vi "Load Becker-Hickl Measurement Descriptions.vi"(6 "Measurement Description Length":i16 format="%.0x", 8 "Error In":errorcluster, 9 "# Measurement Description Blocks":i16 format="%.0x", 10 "Measurement Description Block Offset":i32, 11 "File Path Control":path) -> (0 "Error Out":errorcluster, 2 "Measurement Information":T1 {"Measurement FCS Info"."FCS Type" format="%.0b"; "Measurement FCS Info"."FCS Decay Calc" format="%016b"; "Measurement Stop Info"."Flags" format="%016b"}, 3 "File Path":path)   [LabVIEW 2021, in "Becker-Hickl Files.lvlib"]
uses:
  Becker-Hickl Files.lvlib
  Becker-Hickl Measurement Information.ctl
  Becker-Hickl Measurement Stop Info.ctl
  Becker-Hickl FCS Measurement Info.ctl
  Becker-Hickl Additional Histogram Measurement Info.ctl
  Becker-Hickl Read Single I16.vi
  Becker-Hickl Read Single U16.vi
  Becker-Hickl Read Single U8.vi
  Becker-Hickl Read Single I32.vi
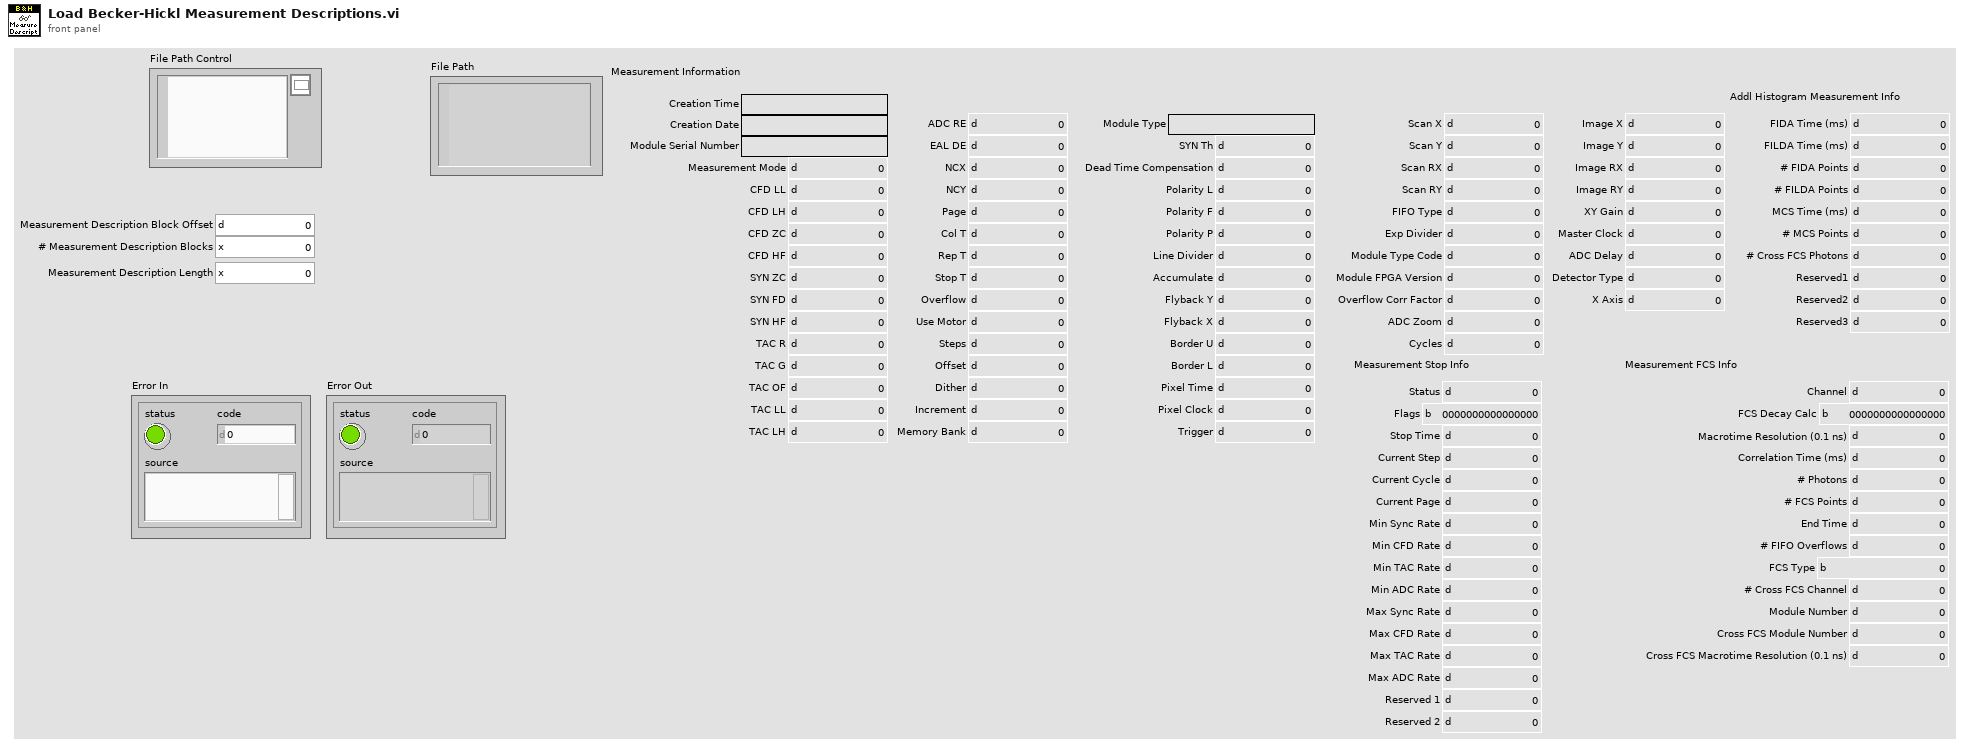
[diagram p1: front panel]
types:
  T1 = typedef "Becker-Hickl Files.lvlib/Becker-Hickl Measurement Information.ctl" = cluster{"Measurement Stop Info":T2, "Measurement FCS Info":T3, "Addl Histogram Measurement Info":T4, "Creation Time":string, "Creation Date":string, "Module Serial Number":string, "Measurement Mode":i16, "CFD LL":sgl, "CFD LH":sgl, "CFD ZC":sgl, "CFD HF":sgl, "SYN ZC":sgl, "SYN FD":i16, "SYN HF":sgl, "TAC R":sgl, "TAC G":i16, "TAC OF":sgl, "TAC LL":sgl, "TAC LH":sgl, "ADC RE":i16, "EAL DE":i16, "NCX":i16, "NCY":i16, "Page":u16, "Col T":sgl, "Rep T":sgl, "Stop T":i16, "Overflow":u8, "Use Motor":i16, "Steps":u16, "Offset":sgl, "Dither":i16, "Increment":i16, "Memory Bank":i16, "Module Type":string, "SYN Th":sgl, "Dead Time Compensation":i16, "Polarity L":i16, "Polarity F":i16, "Polarity P":i16, "Line Divider":i16, "Accumulate":i16, "Flyback Y":i32, "Flyback X":i32, "Border U":i32, "Border L":i32, "Pixel Time":sgl, "Pixel Clock":i16, "Trigger":i16, "Scan X":i32, "Scan Y":i32, "Scan RX":i32, "Scan RY":i32, "FIFO Type":i16, "Exp Divider":i32, "Module Type Code":u16, "Module FPGA Version":u16, "Overflow Corr Factor":sgl, "ADC Zoom":i32, "Cycles":i32, "Image X":i32, "Image Y":i32, "Image RX":i32, "Image RY":i32, "XY Gain":i16, "Master Clock":i16, "ADC Delay":i16, "Detector Type":i16, "X Axis":i16}
  T2 = typedef "Becker-Hickl Files.lvlib/Becker-Hickl Measurement Stop Info.ctl" = cluster{"Status":u16, "Flags":u16, "Stop Time":sgl, "Current Step":i32, "Current Cycle":i32, "Current Page":i32, "Min Sync Rate":sgl, "Min CFD Rate":sgl, "Min TAC Rate":sgl, "Min ADC Rate":sgl, "Max Sync Rate":sgl, "Max CFD Rate":sgl, "Max TAC Rate":sgl, "Max ADC Rate":sgl, "Reserved 1":i32, "Reserved 2":sgl}
  T3 = typedef "Becker-Hickl Files.lvlib/Becker-Hickl FCS Measurement Info.ctl" = cluster{"Channel":u16, "FCS Decay Calc":u16, "Macrotime Resolution (0.1 ns)":u32, "Correlation Time (ms)":sgl, "# Photons":u32, "# FCS Points":i32, "End Time":sgl, "# FIFO Overflows":u16, "FCS Type":u16, "# Cross FCS Channel":u16, "Module Number":u16, "Cross FCS Module Number":u16, "Cross FCS Macrotime Resolution (0.1 ns)":u32}
  T4 = typedef "Becker-Hickl Files.lvlib/Becker-Hickl Additional Histogram Measurement Info.ctl" = cluster{"FIDA Time (ms)":sgl, "FILDA Time (ms)":sgl, "# FIDA Points":i32, "# FILDA Points":i32, "MCS Time (ms)":sgl, "# MCS Points":i32, "# Cross FCS Photons":u32, "Reserved1":i32, "Reserved2":dbl, "Reserved3":dbl}
  T5 = enum16{"time", "date", "mod_ser_no", "meas_mode", "cfd_ll", "cfd_lh", "cfd_zc", "cfd_hf", "syn_zc", "syn_fd", "syn_hf", "tac_r", "tac_g", "tac_of", "tac_ll", "tac_lh", "adc_re", "eal_de", "ncx", "ncy", "page", "col_t", "rep_t", "stopt", "overfl", "use_motor", "steps", "offset", "dither", "incr", "mem_bank", "mod_type", "syn_th", "dead_time_comp", "polarity_l", "polarity_f", "polarity_p", "linediv", "accumulate", "flbck_y", "flbck_x", "bord_u", "bord_l", "pix_time", "pix_clk", "trigger", "scan_x", "scan_y", "scan_rx", "scan_ry", "fifo_typ", "epx_div", "mod_type_code", "mod_fpga_ver", "overflow_corr_factor", "adc_zoom", "cycles", "StopInfo", "FCSInfo", "image_x", "image_y", "image_rx", "image_ry", "xy_gain", "master_clock", "adc_de", "det_type", "x_axis", "HISTInfo"}
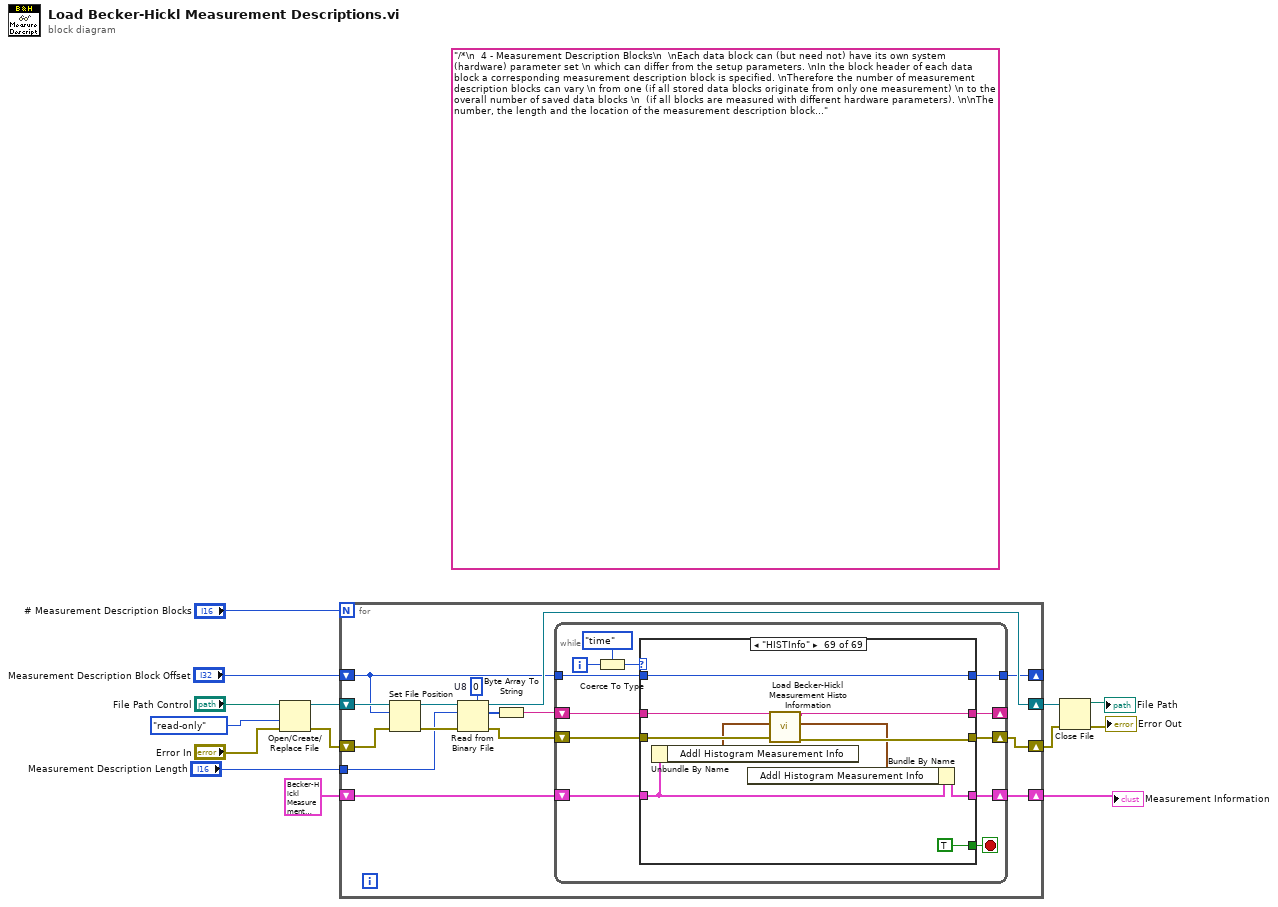
[diagram p0: block diagram]
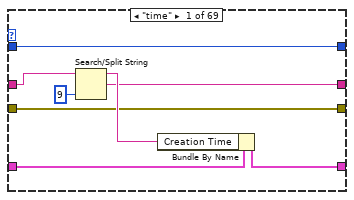
[diagram p2: hidden frame]
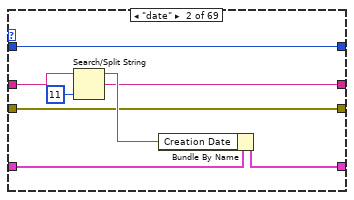
[diagram p3: hidden frame]
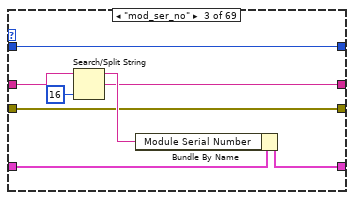
[diagram p4: hidden frame]
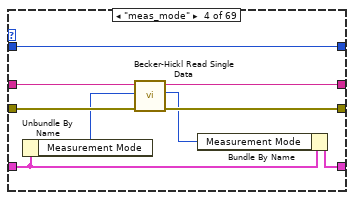
[diagram p5: hidden frame]
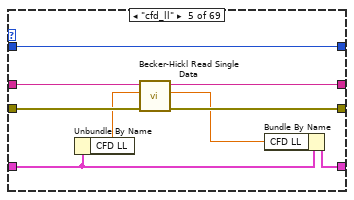
[diagram p6: hidden frame]
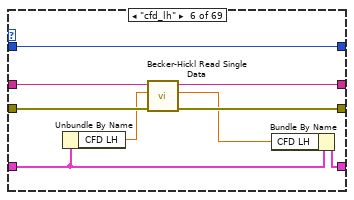
[diagram p7: hidden frame]
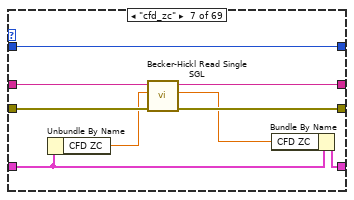
[diagram p8: hidden frame]
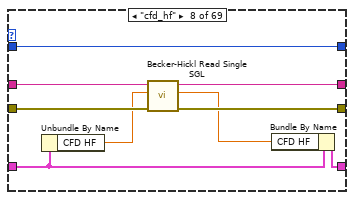
[diagram p9: hidden frame]
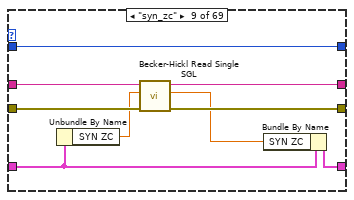
[diagram p10: hidden frame]
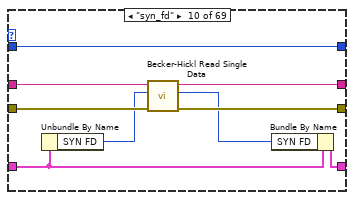
[diagram p11: hidden frame]
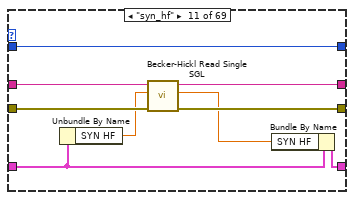
[diagram p12: hidden frame]
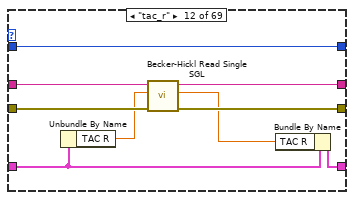
[diagram p13: hidden frame]
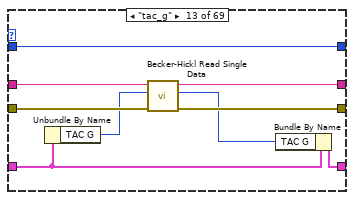
[diagram p14: hidden frame]
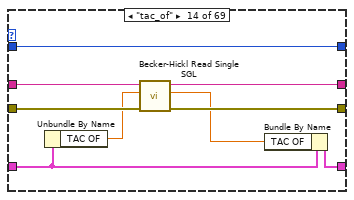
[diagram p15: hidden frame]
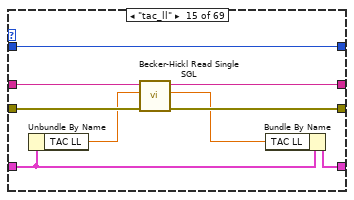
[diagram p16: hidden frame]
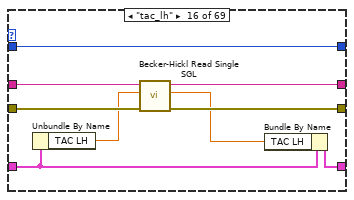
[diagram p17: hidden frame]
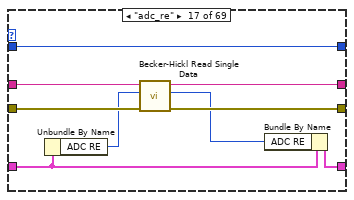
[diagram p18: hidden frame]
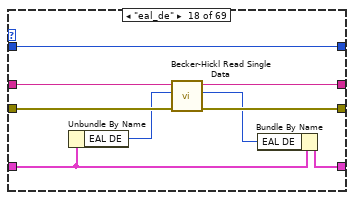
[diagram p19: hidden frame]
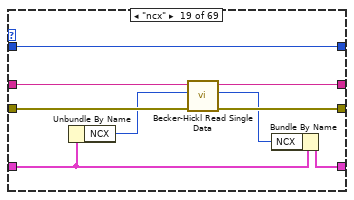
[diagram p20: hidden frame]
diagram:
  (unwired) "/*\n  4 - Measurement Description Blocks\n  \nEach data block can (but need not) have its own system (hardware) parameter set \n which can differ from the setup parameters. \nIn the block header of each data block a corresponding measurement description block is specified. \nTherefore the number of measurement description blocks can vary \n from one (if all stored data blocks originate from only one measurement) \n to the overall number of saved data blocks \n  (if all blocks are measured with different hardware parameters). \n\nThe number, the length and the location of the measurement description blocks is stored \n  in the file header at the beginning of the file.\nThe information in the measurement description blocks is used for \n the 'Block Info' or 'Set Info' function in the Load, Save and Trace Parameters menus. \nIf the button 'Use System Parameters from the Selected Block' is pressed, \n the system parameters are replaced by the data in the measurement description block.\nThe measurement description blocks are stored in a binary format. \n\nFrom the software version 7.9  measurement description block contains also additional \n information (in the structure MeasStopInfo ) collected at the end of the measurement. \n This information can be useful when analyzing system's wrong setup or malfunction.\n\nFrom the software version 8.1  measurement description block contains also additional \n information (in the structure MeasFCSInfo ) collected at the end of the FIFO measurement\n when FCS curve were created.\n The information is valid only for data blocks of type FIFO_DATA or FIFO_DATA_FROM_FILE\n\nFrom the software version 8.3  measurement description block contains also additional \n information (in the structure MeasFIDAInfo ) collected at the end of the FIFO measurement\n when FIDA or FILDA curves were created.\n The information is valid only for data blocks of type FIFO_DATA or FIFO_DATA_FROM_FILE\n\nFrom the software version 8.4  measurement description block contains instead of MeasFIDAInfo\n the structure MeasHISTInfo  collected at the end of the FIFO measurement\n when FIDA , FILDA or MCS curves were created. \n It contains additionally information for MCS curve.\n The information is valid only for data blocks of type FIFO_DATA or FIFO_DATA_FROM_FILE\n\nThe structures are shown below.\n\n*/\n\n\ntypedef struct {\n  unsigned short  status;  // last SPC_test_state return value ( status )\n  unsigned short  flags;   // scan clocks bits 2-0( frame, line, pixel), \n                           //  rates_read - bit 15\n  float  stop_time;        // time from start to  - disarm ( simple measurement )\n                           //    - or to the end of the cycle (for complex measurement )\n  int    cur_step;         // current step  ( if multi-step measurement )\n  int    cur_cycle;        // current cycle (accumulation cycle in FLOW mode ) -\n                           //  ( if multi-cycle measurement ) \n  int    cur_page;         // current measured page\n  float  min_sync_rate;    // minimum rates during the measurement\n  float  min_cfd_rate;     //   ( -1.0 - not set )\n  float  min_tac_rate;\n  float  min_adc_rate;\n  float  max_sync_rate;    // maximum rates during the measurement\n  float  max_cfd_rate;     //   ( -1.0 - not set )\n  float  max_tac_rate;\n  float  max_adc_rate;\n  int    reserved1;\n  float  reserved2;\n  }MeasStopInfo;           // information collected when measurement is finished\n  \n\n\ntypedef struct {\n  unsigned short  chan;               // routing channel number\n  unsigned short  fcs_decay_calc;     // bit 0 = 1 - decay curve calculated\n                                      // bit 1 = 1 - fcs   curve calculated\n                                      // bit 2 = 1 - FIDA  curve calculated\n                                      // bit 3 = 1 - FILDA curve calculated\n                                      // bit 4 = 1 - MCS curve calculated\n                                      // bit 5 = 1 - 3D Image calculated\n  unsigned int    mt_resol;           // macro time clock in 0.1 ns units\n  float           cortime;            // correlation time [ms] \n  unsigned int    calc_photons;       //  no of photons  \n  int             fcs_points;         // no of FCS values\n  float           end_time;           // macro time of the last photon \n  unsigned short  overruns;           // no of Fifo overruns \n                              //   when > 0  fcs curve & end_time are not valid\n  unsigned short  fcs_type;   // 0 - linear FCS with log binning ( 100 bins/log )\n                              // when bit 15 = 1 ( 0x8000 ) - Multi-Tau FCS \n                              //           where bits 14-0 = ktau parameter\n  unsigned short  cross_chan;         // cross FCS routing channel number\n                   //   when chan = cross_chan and mod == cross_mod - Auto FCS\n                   //        otherwise - Cross FCS\n  unsigned short  mod;                // module number\n  unsigned short  cross_mod;          // cross FCS module number\n  unsigned int    cross_mt_resol;     // macro time clock of cross FCS module in 0.1 ns units\n  }MeasFCSInfo;   // information collected when FIFO measurement is finished\n\n\n  \ntypedef struct {\n  float           fida_time;          // interval time [ms] for FIDA histogram\n  float           filda_time;         // interval time [ms] for FILDA histogram\n  int             fida_points;        // no of FIDA values\n                                      //    or current frame number ( fifo_image)\n  int             filda_points;       // no of FILDA values\n                                      //    or current line  number ( fifo_image)\n  float           mcs_time;            // interval time [ms] for MCS histogram\n  int             mcs_points;          // no of MCS values\n                                      //    or current pixel number ( fifo_image)\n  unsigned int    cross_calc_phot;    //  no of calculated photons from cross_channel \n                                      //    for Cross FCS histogram\n  int             reserved1;\n  double          reserved2;\n  double          reserved3;\n  }MeasHISTInfo;     // extension of MeasFCSInfo for other histograms ( FIDA, FILDA, MCS ) \n  \n\ntypedef struct _MeasureInfo {\n  char     time[9];        /* time of creation */\n  char     date[11];       /* date of creation */\n  char     mod_ser_no[16]; /* serial number of the module */\n  short    meas_mode;\n  float    cfd_ll;\n  float    cfd_lh;\n  float    cfd_zc;\n  float    cfd_hf;\n  float    syn_zc;\n  short    syn_fd;\n  float    syn_hf;\n  float    tac_r;\n  short    tac_g;\n  float    tac_of;\n  float    tac_ll;\n  float    tac_lh;\n  short    adc_re;\n  short    eal_de;\n  short    ncx;\n  short    ncy;\n  unsigned short  page;\n  float    col_t;\n  float    rep_t;\n  short    stopt;\n  char     overfl;\n  short    use_motor;\n  unsigned short    steps;\n  float    offset;\n  short    dither;\n  short    incr;\n  short    mem_bank;\n  char     mod_type[16];   /* module type */\n  float    syn_th;\n  short    dead_time_comp;\n  short    polarity_l;   //  2 = disabled line markers\n  short    polarity_f;\n  short    polarity_p;\n  short    linediv;      // line predivider = 2 ** ( linediv)\n  short    accumulate;\n  int      flbck_y; \n  int      flbck_x; \n  int      bord_u; \n  int      bord_l; \n  float    pix_time;\n  short    pix_clk; \n  short    trigger; \n  int      scan_x; \n  int      scan_y; \n  int      scan_rx; \n  int      scan_ry; \n  short    fifo_typ;\n  int      epx_div; \n  unsigned short  mod_type_code; \n  unsigned short  mod_fpga_ver;    // new in v.8.4\n  float    overflow_corr_factor;\n  int      adc_zoom; \n  int      cycles;        //  cycles ( accumulation cycles in FLOW mode ) \n  MeasStopInfo StopInfo;\n  MeasFCSInfo  FCSInfo;   // valid only for FIFO meas\n  int      image_x;       // 4 subsequent fields valid only for Camera mode\n  int      image_y;       //     or FIFO_IMAGE mode\n  int      image_rx; \n  int      image_ry; \n  short    xy_gain;       // gain for XY ADCs ( SPC930 )\n  short    master_clock;  // use or not  Master Clock (SPC140 multi-module )\n  short    adc_de;        // ADC sample delay ( SPC-930 )\n  short    det_type;      // detector type ( SPC-930 in camera mode ) \n  short    x_axis;        // X axis representation ( SPC-930 ) \n  MeasHISTInfo  HISTInfo; // extension of FCSInfo, valid only for FIFO meas\n  }MeasureInfo;\n\n"
  n1 = Open/Create/Replace File(file path (use dialog)="File Path Control", error in="Error In", access (0:read/write)=enum16{"read/write", "read-only", "write-only"}."read-only") -> (refnum out=w11:refnum<file>, error out=w10:errorcluster)  [unwired: 3 in, 1 out]
  n2 = for {
    N: "# Measurement Description Blocks" -> [_]
    shift-right: [w23] -> w7
    shift-left: w10 -> [w26]
    shift-right: [w21] -> w8
    shift-left: w11 -> [w27]
    shift-right: [w20] -> _
    shift-left: "Measurement Description Block Offset" -> [w19]
    tunnel: "Measurement Description Length" -> [w18]
    shift-right: [w16] -> w1
    shift-left: T1 {"Measurement Stop Info"={"Status"=0, "Flags"=0, "Stop Time"=0.0, "Current Step"=0, "Current Cycle"=0, "Current Page"=0, "Min Sync Rate"=0.0, "Min CFD Rate"=0.0, "Min TAC Rate"=0.0, "Min ADC Rate"=0.0, "Max Sync Rate"=0.0, "Max CFD Rate"=0.0, "Max TAC Rate"=0.0, "Max ADC Rate"=0.0, "Reserved 1"=0, "Reserved 2"=0.0}, "Measurement FCS Info"={"Channel"=0, "FCS Decay Calc"=0, "Macrotime Resolution (0.1 ns)"=0, "Correlation Time (ms)"=0.0, "# Photons"=0, "# FCS Points"=0, "End Time"=0.0, "# FIFO Overflows"=0, "FCS Type"=0, "# Cross FCS Channel"=0, "Module Number"=0, "Cross FCS Module Number"=0, "Cross FCS Macrotime Resolution (0.1 ns)"=0}, "Addl Histogram Measurement Info"={"FIDA Time (ms)"=0.0, "FILDA Time (ms)"=0.0, "# FIDA Points"=0, "# FILDA Points"=0, "MCS Time (ms)"=0.0, "# MCS Points"=0, "# Cross FCS Photons"=0, "Reserved1"=0, "Reserved2"=0.0, "Reserved3"=0.0}, "Creation Time"="", "Creation Date"="", "Module Serial Number"="", "Measurement Mode"=0, "CFD LL"=0.0, "CFD LH"=0.0, "CFD ZC"=0.0, "CFD HF"=0.0, "SYN ZC"=0.0, "SYN FD"=0, "SYN HF"=0.0, "TAC R"=0.0, "TAC G"=0, "TAC OF"=0.0, "TAC LL"=0.0, "TAC LH"=0.0, "ADC RE"=0, "EAL DE"=0, "NCX"=0, "NCY"=0, "Page"=0, "Col T"=0.0, "Rep T"=0.0, "Stop T"=0, "Overflow"=0, "Use Motor"=0, "Steps"=0, "Offset"=0.0, "Dither"=0, "Increment"=0, "Memory Bank"=0, "Module Type"="", "SYN Th"=0.0, "Dead Time Compensation"=0, "Polarity L"=0, "Polarity F"=0, "Polarity P"=0, "Line Divider"=0, "Accumulate"=0, "Flyback Y"=0, "Flyback X"=0, "Border U"=0, "Border L"=0, "Pixel Time"=0.0, "Pixel Clock"=0, "Trigger"=0, "Scan X"=0, "Scan Y"=0, "Scan RX"=0, "Scan RY"=0, "FIFO Type"=0, "Exp Divider"=0, "Module Type Code"=0, "Module FPGA Version"=0, "Overflow Corr Factor"=0.0, "ADC Zoom"=0, "Cycles"=0, "Image X"=0, "Image Y"=0, "Image RX"=0, "Image RY"=0, "XY Gain"=0, "Master Clock"=0, "ADC Delay"=0, "Detector Type"=0, "X Axis"=0} ("Measurement Information") -> [w17]
    w29 = u8 0  # U8
    n3 = Set File Position(offset (in bytes) (0)=w19, refnum=w27, error in=w26) -> (refnum out=w25:refnum<file>, error out=w24:errorcluster)  [unwired: 1 in]
    n4 = Read from Binary File(5:w29, 8:w24, 10:w18, 11:w25) -> (0:w22:errorcluster, 2:w28:u8[], 3:w21:refnum<file>)  [unwired: 2 in, 1 out]
    n5 = Byte Array To String(unsigned byte array=w28) -> (string=w15:string)
    n6 = while {
      shift-right: [w36] -> w23
      shift-left: w22 -> [w40]
      shift-right: [w35] -> _
      shift-left: w15 -> [w39]
      shift-right: [w37] -> w16
      shift-left: w17 -> [w38]
      tunnel: [w34] -> w20
      tunnel: w19 -> [w33]
      i -> [w41]
      stop <- w30 stop-if-true
      n7 = Coerce To Type(0:w41, 1:T5."time") -> (2:w32:T5)
      n8 = case shown="\"HISTInfo\"" w32 {
        tunnel: w40 -> [w42 w50 w58 w71 w80 w89 w98 w107 w116 w125 w134 w143 w152 w161 w170 w179 w188 w197 w206 w215 w224 w233 w242 w251 w260 w269 w278 w287 w296 w305 w314 w321 w331 w340 w349 w358 w367 w376 w385 w394 w403 w412 w421 w430 w439 w448 w457 w466 w475 w484 w493 w502 w511 w520 w529 w538 w547 w554 w563 w574 w583 w592 w601 w610 w619 w628 w637 w646 w654]
        tunnel: w39 -> [w46 w54 w62 w72 w81 w90 w99 w108 w117 w126 w135 w144 w153 w162 w171 w180 w189 w198 w207 w216 w225 w234 w243 w252 w261 w270 w279 w288 w297 w306 w315 w322 w332 w341 w350 w359 w368 w377 w386 w395 w404 w413 w422 w431 w440 w449 w458 w467 w476 w485 w494 w503 w512 w521 w530 w539 w548 w556 w565 w575 w584 w593 w602 w611 w620 w629 w638 w647 w655]
        tunnel: w38 -> [w48 w56 w64 w67 w76 w85 w94 w103 w112 w121 w130 w139 w148 w157 w166 w175 w184 w193 w202 w211 w220 w229 w238 w247 w256 w265 w274 w283 w292 w301 w310 w323 w327 w336 w345 w354 w363 w372 w381 w390 w399 w408 w417 w426 w435 w444 w453 w462 w471 w480 w489 w498 w507 w516 w525 w534 w543 w557 w566 w570 w579 w588 w597 w606 w615 w624 w633 w642 w657]
        tunnel: [w47 w55 w63 w73 w82 w91 w100 w109 w118 w127 w136 w145 w154 w163 w172 w181 w190 w199 w208 w217 w226 w235 w244 w253 w262 w271 w280 w289 w298 w307 w316 w324 w333 w342 w351 w360 w369 w378 w387 w396 w405 w414 w423 w432 w441 w450 w459 w468 w477 w486 w495 w504 w513 w522 w531 w540 w549 w558 w567 w576 w585 w594 w603 w612 w621 w630 w639 w648 w658] -> w37
        tunnel: [w42 w50 w58 w70 w79 w88 w97 w106 w115 w124 w133 w142 w151 w160 w169 w178 w187 w196 w205 w214 w223 w232 w241 w250 w259 w268 w277 w286 w295 w304 w313 w321 w330 w339 w348 w357 w366 w375 w384 w393 w402 w411 w420 w429 w438 w447 w456 w465 w474 w483 w492 w501 w510 w519 w528 w537 w546 w553 w562 w573 w582 w591 w600 w609 w618 w627 w636 w645 w652] -> w36
        tunnel: [w43 w51 w59 w69 w78 w87 w96 w105 w114 w123 w132 w141 w150 w159 w168 w177 w186 w195 w204 w213 w222 w231 w240 w249 w258 w267 w276 w285 w294 w303 w312 w319 w329 w338 w347 w356 w365 w374 w383 w392 w401 w410 w419 w428 w437 w446 w455 w464 w473 w482 w491 w500 w509 w518 w527 w536 w545 w555 w564 w572 w581 w590 w599 w608 w617 w626 w635 w644 w653] -> w35
        tunnel: [w49 w57 w65 w74 w83 w92 w101 w110 w119 w128 w137 w146 w155 w164 w173 w182 w191 w200 w209 w218 w227 w236 w245 w254 w263 w272 w281 w290 w299 w308 w317 w325 w334 w343 w352 w361 w370 w379 w388 w397 w406 w415 w424 w433 w442 w451 w460 w469 w478 w487 w496 w505 w514 w523 w532 w541 w550 w559 w568 w577 w586 w595 w604 w613 w622 w631 w640 w649 w659] -> w34
        tunnel: w33 -> [w49 w57 w65 w74 w83 w92 w101 w110 w119 w128 w137 w146 w155 w164 w173 w182 w191 w200 w209 w218 w227 w236 w245 w254 w263 w272 w281 w290 w299 w308 w317 w325 w334 w343 w352 w361 w370 w379 w388 w397 w406 w415 w424 w433 w442 w451 w460 w469 w478 w487 w496 w505 w514 w523 w532 w541 w550 w559 w568 w577 w586 w595 w604 w613 w622 w631 w640 w649 w659]
        tunnel: [_ _ _ _ _ _ _ _ _ _ _ _ _ _ _ _ _ _ _ _ _ _ _ _ _ _ _ _ _ _ _ _ _ _ _ _ _ _ _ _ _ _ _ _ _ _ _ _ _ _ _ _ _ _ _ _ _ _ _ _ _ _ _ _ _ _ _ _ TRUE] -> w30
        frame "time" {
          n9 = Search/Split String(string=w46, offset (0)=9) -> (substring before match=w44:string, match + rest of string=w43:string)  [unwired: 1 in, 1 out]
          n10 = Bundle By Name(cluster=w48, "Creation Time"=w44) -> (w47:T1)
        }
        frame "date" {
          n11 = Search/Split String(string=w54, offset (0)=11) -> (substring before match=w52:string, match + rest of string=w51:string)  [unwired: 1 in, 1 out]
          n12 = Bundle By Name(cluster=w56, "Creation Date"=w52) -> (w55:T1)
        }
        frame "mod_ser_no" {
          n13 = Search/Split String(string=w62, offset (0)=16) -> (substring before match=w60:string, match + rest of string=w59:string)  [unwired: 1 in, 1 out]
          n14 = Bundle By Name(cluster=w64, "Module Serial Number"=w60) -> (w63:T1)
        }
        frame "meas_mode" {
          n15 = Unbundle By Name(w67) -> ("Measurement Mode"=w66:i16)
          n16 = call-poly "Becker-Hickl Read Single Data.vi"("Error In"=w71, "Default"=w66, "Bytes in"=w72) -> ("Error Out"=w70:errorcluster, "I16"=w68:i16, "Bytes out"=w69:string)  [unwired: 6 in]
          n17 = Bundle By Name(cluster=w67, "Measurement Mode"=w68) -> (w73:T1)
        }
        frame "cfd_ll" {
          n18 = Unbundle By Name(w76) -> ("CFD LL"=w75:sgl)
          n19 = call-poly "Becker-Hickl Read Single Data.vi"("Error In"=w80, "Default"=w75, "Bytes in"=w81) -> ("Error Out"=w79:errorcluster, "SGL"=w77:sgl, "Bytes out"=w78:string)  [unwired: 6 in]
          n20 = Bundle By Name(cluster=w76, "CFD LL"=w77) -> (w82:T1)
        }
        frame "cfd_lh" {
          n21 = Unbundle By Name(w85) -> ("CFD LH"=w84:sgl)
          n22 = call-poly "Becker-Hickl Read Single Data.vi"("Error In"=w89, "Default"=w84, "Bytes in"=w90) -> ("Error Out"=w88:errorcluster, "SGL"=w86:sgl, "Bytes out"=w87:string)  [unwired: 6 in]
          n23 = Bundle By Name(cluster=w85, "CFD LH"=w86) -> (w91:T1)
        }
        frame "cfd_zc" {
          n24 = Unbundle By Name(w94) -> ("CFD ZC"=w93:sgl)
          n25 = call "Becker-Hickl Read Single SGL.vi"("Error In"=w98, "Default"=w93, "Bytes in"=w99) -> ("Error Out"=w97:errorcluster, "SGL"=w95:sgl, "Bytes out"=w96:string)  [unwired: 6 in]
          n26 = Bundle By Name(cluster=w94, "CFD ZC"=w95) -> (w100:T1)
        }
        frame "cfd_hf" {
          n27 = Unbundle By Name(w103) -> ("CFD HF"=w102:sgl)
          n28 = call "Becker-Hickl Read Single SGL.vi"("Error In"=w107, "Default"=w102, "Bytes in"=w108) -> ("Error Out"=w106:errorcluster, "SGL"=w104:sgl, "Bytes out"=w105:string)  [unwired: 6 in]
          n29 = Bundle By Name(cluster=w103, "CFD HF"=w104) -> (w109:T1)
        }
        frame "syn_zc" {
          n30 = Unbundle By Name(w112) -> ("SYN ZC"=w111:sgl)
          n31 = call "Becker-Hickl Read Single SGL.vi"("Error In"=w116, "Default"=w111, "Bytes in"=w117) -> ("Error Out"=w115:errorcluster, "SGL"=w113:sgl, "Bytes out"=w114:string)  [unwired: 6 in]
          n32 = Bundle By Name(cluster=w112, "SYN ZC"=w113) -> (w118:T1)
        }
        frame "syn_fd" {
          n33 = Unbundle By Name(w121) -> ("SYN FD"=w120:i16)
          n34 = call-poly "Becker-Hickl Read Single Data.vi"("Error In"=w125, "Default"=w120, "Bytes in"=w126) -> ("Error Out"=w124:errorcluster, "I16"=w122:i16, "Bytes out"=w123:string)  [unwired: 6 in]
          n35 = Bundle By Name(cluster=w121, "SYN FD"=w122) -> (w127:T1)
        }
        frame "syn_hf" {
          n36 = Unbundle By Name(w130) -> ("SYN HF"=w129:sgl)
          n37 = call "Becker-Hickl Read Single SGL.vi"("Error In"=w134, "Default"=w129, "Bytes in"=w135) -> ("Error Out"=w133:errorcluster, "SGL"=w131:sgl, "Bytes out"=w132:string)  [unwired: 6 in]
          n38 = Bundle By Name(cluster=w130, "SYN HF"=w131) -> (w136:T1)
        }
        frame "tac_r" {
          n39 = Unbundle By Name(w139) -> ("TAC R"=w138:sgl)
          n40 = call "Becker-Hickl Read Single SGL.vi"("Error In"=w143, "Default"=w138, "Bytes in"=w144) -> ("Error Out"=w142:errorcluster, "SGL"=w140:sgl, "Bytes out"=w141:string)  [unwired: 6 in]
          n41 = Bundle By Name(cluster=w139, "TAC R"=w140) -> (w145:T1)
        }
        frame "tac_g" {
          n42 = Unbundle By Name(w148) -> ("TAC G"=w147:i16)
          n43 = call-poly "Becker-Hickl Read Single Data.vi"("Error In"=w152, "Default"=w147, "Bytes in"=w153) -> ("Error Out"=w151:errorcluster, "I16"=w149:i16, "Bytes out"=w150:string)  [unwired: 6 in]
          n44 = Bundle By Name(cluster=w148, "TAC G"=w149) -> (w154:T1)
        }
        frame "tac_of" {
          n45 = Unbundle By Name(w157) -> ("TAC OF"=w156:sgl)
          n46 = call "Becker-Hickl Read Single SGL.vi"("Error In"=w161, "Default"=w156, "Bytes in"=w162) -> ("Error Out"=w160:errorcluster, "SGL"=w158:sgl, "Bytes out"=w159:string)  [unwired: 6 in]
          n47 = Bundle By Name(cluster=w157, "TAC OF"=w158) -> (w163:T1)
        }
        frame "tac_ll" {
          n48 = Unbundle By Name(w166) -> ("TAC LL"=w165:sgl)
          n49 = call "Becker-Hickl Read Single SGL.vi"("Error In"=w170, "Default"=w165, "Bytes in"=w171) -> ("Error Out"=w169:errorcluster, "SGL"=w167:sgl, "Bytes out"=w168:string)  [unwired: 6 in]
          n50 = Bundle By Name(cluster=w166, "TAC LL"=w167) -> (w172:T1)
        }
        frame "tac_lh" {
          n51 = Unbundle By Name(w175) -> ("TAC LH"=w174:sgl)
          n52 = call "Becker-Hickl Read Single SGL.vi"("Error In"=w179, "Default"=w174, "Bytes in"=w180) -> ("Error Out"=w178:errorcluster, "SGL"=w176:sgl, "Bytes out"=w177:string)  [unwired: 6 in]
          n53 = Bundle By Name(cluster=w175, "TAC LH"=w176) -> (w181:T1)
        }
        frame "adc_re" {
          n54 = Unbundle By Name(w184) -> ("ADC RE"=w183:i16)
          n55 = call-poly "Becker-Hickl Read Single Data.vi"("Error In"=w188, "Default"=w183, "Bytes in"=w189) -> ("Error Out"=w187:errorcluster, "I16"=w185:i16, "Bytes out"=w186:string)  [unwired: 6 in]
          n56 = Bundle By Name(cluster=w184, "ADC RE"=w185) -> (w190:T1)
        }
        frame "eal_de" {
          n57 = Unbundle By Name(w193) -> ("EAL DE"=w192:i16)
          n58 = call-poly "Becker-Hickl Read Single Data.vi"("Error In"=w197, "Default"=w192, "Bytes in"=w198) -> ("Error Out"=w196:errorcluster, "I16"=w194:i16, "Bytes out"=w195:string)  [unwired: 6 in]
          n59 = Bundle By Name(cluster=w193, "EAL DE"=w194) -> (w199:T1)
        }
        frame "ncx" {
          n60 = Unbundle By Name(w202) -> ("NCX"=w201:i16)
          n61 = call-poly "Becker-Hickl Read Single Data.vi"("Error In"=w206, "Default"=w201, "Bytes in"=w207) -> ("Error Out"=w205:errorcluster, "I16"=w203:i16, "Bytes out"=w204:string)  [unwired: 6 in]
          n62 = Bundle By Name(cluster=w202, "NCX"=w203) -> (w208:T1)
        }
        frame "ncy" {
          n63 = Unbundle By Name(w211) -> ("NCY"=w210:i16)
          n64 = call-poly "Becker-Hickl Read Single Data.vi"("Error In"=w215, "Default"=w210, "Bytes in"=w216) -> ("Error Out"=w214:errorcluster, "I16"=w212:i16, "Bytes out"=w213:string)  [unwired: 6 in]
          n65 = Bundle By Name(cluster=w211, "NCY"=w212) -> (w217:T1)
        }
        frame "page" {
          n66 = Unbundle By Name(w220) -> ("Page"=w219:u16)
          n67 = call-poly "Becker-Hickl Read Single Data.vi"("Error In"=w224, "Default"=w219, "Bytes in"=w225) -> ("Error Out"=w223:errorcluster, "U16"=w221:u16, "Bytes out"=w222:string)  [unwired: 6 in]
          n68 = Bundle By Name(cluster=w220, "Page"=w221) -> (w226:T1)
        }
        frame "col_t" {
          n69 = Unbundle By Name(w229) -> ("Col T"=w228:sgl)
          n70 = call "Becker-Hickl Read Single SGL.vi"("Error In"=w233, "Default"=w228, "Bytes in"=w234) -> ("Error Out"=w232:errorcluster, "SGL"=w230:sgl, "Bytes out"=w231:string)  [unwired: 6 in]
          n71 = Bundle By Name(cluster=w229, "Col T"=w230) -> (w235:T1)
        }
        frame "rep_t" {
          n72 = Unbundle By Name(w238) -> ("Rep T"=w237:sgl)
          n73 = call "Becker-Hickl Read Single SGL.vi"("Error In"=w242, "Default"=w237, "Bytes in"=w243) -> ("Error Out"=w241:errorcluster, "SGL"=w239:sgl, "Bytes out"=w240:string)  [unwired: 6 in]
          n74 = Bundle By Name(cluster=w238, "Rep T"=w239) -> (w244:T1)
        }
        frame "stopt" {
          n75 = Unbundle By Name(w247) -> ("Stop T"=w246:i16)
          n76 = call-poly "Becker-Hickl Read Single Data.vi"("Error In"=w251, "Default"=w246, "Bytes in"=w252) -> ("Error Out"=w250:errorcluster, "I16"=w248:i16, "Bytes out"=w249:string)  [unwired: 6 in]
          n77 = Bundle By Name(cluster=w247, "Stop T"=w248) -> (w253:T1)
        }
        frame "overfl" {
          n78 = Unbundle By Name(w256) -> ("Overflow"=w255:u8)
          n79 = call-poly "Becker-Hickl Read Single Data.vi"("Error In"=w260, "Default"=w255, "Bytes in"=w261) -> ("Error Out"=w259:errorcluster, "U8"=w257:u8, "Bytes out"=w258:string)  [unwired: 6 in]
          n80 = Bundle By Name(cluster=w256, "Overflow"=w257) -> (w262:T1)
        }
        frame "use_motor" {
          n81 = Unbundle By Name(w265) -> ("Use Motor"=w264:i16)
          n82 = call-poly "Becker-Hickl Read Single Data.vi"("Error In"=w269, "Default"=w264, "Bytes in"=w270) -> ("Error Out"=w268:errorcluster, "I16"=w266:i16, "Bytes out"=w267:string)  [unwired: 6 in]
          n83 = Bundle By Name(cluster=w265, "Use Motor"=w266) -> (w271:T1)
        }
        frame "steps" {
          n84 = Unbundle By Name(w274) -> ("Steps"=w273:u16)
          n85 = call-poly "Becker-Hickl Read Single Data.vi"("Error In"=w278, "Default"=w273, "Bytes in"=w279) -> ("Error Out"=w277:errorcluster, "U16"=w275:u16, "Bytes out"=w276:string)  [unwired: 6 in]
          n86 = Bundle By Name(cluster=w274, "Steps"=w275) -> (w280:T1)
        }
        frame "offset" {
          n87 = Unbundle By Name(w283) -> ("Offset"=w282:sgl)
          n88 = call-poly "Becker-Hickl Read Single Data.vi"("Error In"=w287, "Default"=w282, "Bytes in"=w288) -> ("Error Out"=w286:errorcluster, "SGL"=w284:sgl, "Bytes out"=w285:string)  [unwired: 6 in]
          n89 = Bundle By Name(cluster=w283, "Offset"=w284) -> (w289:T1)
        }
        frame "dither" {
          n90 = Unbundle By Name(w292) -> ("Dither"=w291:i16)
          n91 = call-poly "Becker-Hickl Read Single Data.vi"("Error In"=w296, "Default"=w291, "Bytes in"=w297) -> ("Error Out"=w295:errorcluster, "I16"=w293:i16, "Bytes out"=w294:string)  [unwired: 6 in]
          n92 = Bundle By Name(cluster=w292, "Dither"=w293) -> (w298:T1)
        }
        frame "incr" {
          n93 = Unbundle By Name(w301) -> ("Increment"=w300:i16)
          n94 = call-poly "Becker-Hickl Read Single Data.vi"("Error In"=w305, "Default"=w300, "Bytes in"=w306) -> ("Error Out"=w304:errorcluster, "I16"=w302:i16, "Bytes out"=w303:string)  [unwired: 6 in]
          n95 = Bundle By Name(cluster=w301, "Increment"=w302) -> (w307:T1)
        }
        frame "mem_bank" {
          n96 = Unbundle By Name(w310) -> ("Memory Bank"=w309:i16)
          n97 = call-poly "Becker-Hickl Read Single Data.vi"("Error In"=w314, "Default"=w309, "Bytes in"=w315) -> ("Error Out"=w313:errorcluster, "I16"=w311:i16, "Bytes out"=w312:string)  [unwired: 6 in]
          n98 = Bundle By Name(cluster=w310, "Memory Bank"=w311) -> (w316:T1)
        }
        frame "mod_type" {
          n99 = Search/Split String(string=w322, offset (0)=16) -> (substring before match=w320:string, match + rest of string=w319:string)  [unwired: 1 in, 1 out]
          n100 = Bundle By Name(cluster=w323, "Module Type"=w320) -> (w324:T1)
        }
        frame "syn_th" {
          n101 = Unbundle By Name(w327) -> ("SYN Th"=w326:sgl)
          n102 = call-poly "Becker-Hickl Read Single Data.vi"("Error In"=w331, "Default"=w326, "Bytes in"=w332) -> ("Error Out"=w330:errorcluster, "SGL"=w328:sgl, "Bytes out"=w329:string)  [unwired: 6 in]
          n103 = Bundle By Name(cluster=w327, "SYN Th"=w328) -> (w333:T1)
        }
        frame "dead_time_comp" {
          n104 = Unbundle By Name(w336) -> ("Dead Time Compensation"=w335:i16)
          n105 = call-poly "Becker-Hickl Read Single Data.vi"("Error In"=w340, "Default"=w335, "Bytes in"=w341) -> ("Error Out"=w339:errorcluster, "I16"=w337:i16, "Bytes out"=w338:string)  [unwired: 6 in]
          n106 = Bundle By Name(cluster=w336, "Dead Time Compensation"=w337) -> (w342:T1)
        }
        frame "polarity_l" {
          n107 = Unbundle By Name(w345) -> ("Polarity L"=w344:i16)
          n108 = call-poly "Becker-Hickl Read Single Data.vi"("Error In"=w349, "Default"=w344, "Bytes in"=w350) -> ("Error Out"=w348:errorcluster, "I16"=w346:i16, "Bytes out"=w347:string)  [unwired: 6 in]
          n109 = Bundle By Name(cluster=w345, "Polarity L"=w346) -> (w351:T1)
        }
        frame "polarity_f" {
          n110 = Unbundle By Name(w354) -> ("Polarity F"=w353:i16)
          n111 = call-poly "Becker-Hickl Read Single Data.vi"("Error In"=w358, "Default"=w353, "Bytes in"=w359) -> ("Error Out"=w357:errorcluster, "I16"=w355:i16, "Bytes out"=w356:string)  [unwired: 6 in]
          n112 = Bundle By Name(cluster=w354, "Polarity F"=w355) -> (w360:T1)
        }
        frame "polarity_p" {
          n113 = Unbundle By Name(w363) -> ("Polarity P"=w362:i16)
          n114 = call-poly "Becker-Hickl Read Single Data.vi"("Error In"=w367, "Default"=w362, "Bytes in"=w368) -> ("Error Out"=w366:errorcluster, "I16"=w364:i16, "Bytes out"=w365:string)  [unwired: 6 in]
          n115 = Bundle By Name(cluster=w363, "Polarity P"=w364) -> (w369:T1)
        }
        frame "linediv" {
          n116 = Unbundle By Name(w372) -> ("Line Divider"=w371:i16)
          n117 = call-poly "Becker-Hickl Read Single Data.vi"("Error In"=w376, "Default"=w371, "Bytes in"=w377) -> ("Error Out"=w375:errorcluster, "I16"=w373:i16, "Bytes out"=w374:string)  [unwired: 6 in]
          n118 = Bundle By Name(cluster=w372, "Line Divider"=w373) -> (w378:T1)
        }
        frame "accumulate" {
          n119 = Unbundle By Name(w381) -> ("Accumulate"=w380:i16)
          n120 = call-poly "Becker-Hickl Read Single Data.vi"("Error In"=w385, "Default"=w380, "Bytes in"=w386) -> ("Error Out"=w384:errorcluster, "I16"=w382:i16, "Bytes out"=w383:string)  [unwired: 6 in]
          n121 = Bundle By Name(cluster=w381, "Accumulate"=w382) -> (w387:T1)
        }
        frame "flbck_y" {
          n122 = Unbundle By Name(w390) -> ("Flyback Y"=w389:i32)
          n123 = call-poly "Becker-Hickl Read Single Data.vi"("Error In"=w394, "Default"=w389, "Bytes in"=w395) -> ("Error Out"=w393:errorcluster, "I32"=w391:i32, "Bytes out"=w392:string)  [unwired: 6 in]
          n124 = Bundle By Name(cluster=w390, "Flyback Y"=w391) -> (w396:T1)
        }
        frame "flbck_x" {
          n125 = Unbundle By Name(w399) -> ("Flyback X"=w398:i32)
          n126 = call-poly "Becker-Hickl Read Single Data.vi"("Error In"=w403, "Default"=w398, "Bytes in"=w404) -> ("Error Out"=w402:errorcluster, "I32"=w400:i32, "Bytes out"=w401:string)  [unwired: 6 in]
          n127 = Bundle By Name(cluster=w399, "Flyback X"=w400) -> (w405:T1)
        }
        frame "bord_u" {
          n128 = Unbundle By Name(w408) -> ("Border U"=w407:i32)
          n129 = call-poly "Becker-Hickl Read Single Data.vi"("Error In"=w412, "Default"=w407, "Bytes in"=w413) -> ("Error Out"=w411:errorcluster, "I32"=w409:i32, "Bytes out"=w410:string)  [unwired: 6 in]
          n130 = Bundle By Name(cluster=w408, "Border U"=w409) -> (w414:T1)
        }
        frame "bord_l" {
          n131 = Unbundle By Name(w417) -> ("Border L"=w416:i32)
          n132 = call-poly "Becker-Hickl Read Single Data.vi"("Error In"=w421, "Default"=w416, "Bytes in"=w422) -> ("Error Out"=w420:errorcluster, "I32"=w418:i32, "Bytes out"=w419:string)  [unwired: 6 in]
          n133 = Bundle By Name(cluster=w417, "Border L"=w418) -> (w423:T1)
        }
        frame "pix_time" {
          n134 = Unbundle By Name(w426) -> ("Pixel Time"=w425:sgl)
          n135 = call-poly "Becker-Hickl Read Single Data.vi"("Error In"=w430, "Default"=w425, "Bytes in"=w431) -> ("Error Out"=w429:errorcluster, "SGL"=w427:sgl, "Bytes out"=w428:string)  [unwired: 6 in]
          n136 = Bundle By Name(cluster=w426, "Pixel Time"=w427) -> (w432:T1)
        }
        frame "pix_clk" {
          n137 = Unbundle By Name(w435) -> ("Pixel Clock"=w434:i16)
          n138 = call-poly "Becker-Hickl Read Single Data.vi"("Error In"=w439, "Default"=w434, "Bytes in"=w440) -> ("Error Out"=w438:errorcluster, "I16"=w436:i16, "Bytes out"=w437:string)  [unwired: 6 in]
          n139 = Bundle By Name(cluster=w435, "Pixel Clock"=w436) -> (w441:T1)
        }
        frame "trigger" {
          n140 = Unbundle By Name(w444) -> ("Trigger"=w443:i16)
          n141 = call-poly "Becker-Hickl Read Single Data.vi"("Error In"=w448, "Default"=w443, "Bytes in"=w449) -> ("Error Out"=w447:errorcluster, "I16"=w445:i16, "Bytes out"=w446:string)  [unwired: 6 in]
          n142 = Bundle By Name(cluster=w444, "Trigger"=w445) -> (w450:T1)
        }
        frame "scan_x" {
          n143 = Unbundle By Name(w453) -> ("Scan X"=w452:i32)
          n144 = call-poly "Becker-Hickl Read Single Data.vi"("Error In"=w457, "Default"=w452, "Bytes in"=w458) -> ("Error Out"=w456:errorcluster, "I32"=w454:i32, "Bytes out"=w455:string)  [unwired: 6 in]
          n145 = Bundle By Name(cluster=w453, "Scan X"=w454) -> (w459:T1)
        }
        frame "scan_y" {
          n146 = Unbundle By Name(w462) -> ("Scan Y"=w461:i32)
          n147 = call-poly "Becker-Hickl Read Single Data.vi"("Error In"=w466, "Default"=w461, "Bytes in"=w467) -> ("Error Out"=w465:errorcluster, "I32"=w463:i32, "Bytes out"=w464:string)  [unwired: 6 in]
          n148 = Bundle By Name(cluster=w462, "Scan Y"=w463) -> (w468:T1)
        }
        frame "scan_rx" {
          n149 = Unbundle By Name(w471) -> ("Scan RX"=w470:i32)
          n150 = call-poly "Becker-Hickl Read Single Data.vi"("Error In"=w475, "Default"=w470, "Bytes in"=w476) -> ("Error Out"=w474:errorcluster, "I32"=w472:i32, "Bytes out"=w473:string)  [unwired: 6 in]
          n151 = Bundle By Name(cluster=w471, "Scan RX"=w472) -> (w477:T1)
        }
        frame "scan_ry" {
          n152 = Unbundle By Name(w480) -> ("Scan RY"=w479:i32)
          n153 = call-poly "Becker-Hickl Read Single Data.vi"("Error In"=w484, "Default"=w479, "Bytes in"=w485) -> ("Error Out"=w483:errorcluster, "I32"=w481:i32, "Bytes out"=w482:string)  [unwired: 6 in]
          n154 = Bundle By Name(cluster=w480, "Scan RY"=w481) -> (w486:T1)
        }
        frame "fifo_typ" {
          n155 = Unbundle By Name(w489) -> ("FIFO Type"=w488:i16)
          n156 = call-poly "Becker-Hickl Read Single Data.vi"("Error In"=w493, "Default"=w488, "Bytes in"=w494) -> ("Error Out"=w492:errorcluster, "I16"=w490:i16, "Bytes out"=w491:string)  [unwired: 6 in]
          n157 = Bundle By Name(cluster=w489, "FIFO Type"=w490) -> (w495:T1)
        }
        frame "epx_div" {
          n158 = Unbundle By Name(w498) -> ("Exp Divider"=w497:i32)
          n159 = call-poly "Becker-Hickl Read Single Data.vi"("Error In"=w502, "Default"=w497, "Bytes in"=w503) -> ("Error Out"=w501:errorcluster, "I32"=w499:i32, "Bytes out"=w500:string)  [unwired: 6 in]
          n160 = Bundle By Name(cluster=w498, "Exp Divider"=w499) -> (w504:T1)
        }
        frame "mod_type_code" {
          n161 = Unbundle By Name(w507) -> ("Module Type Code"=w506:u16)
          n162 = call-poly "Becker-Hickl Read Single Data.vi"("Error In"=w511, "Default"=w506, "Bytes in"=w512) -> ("Error Out"=w510:errorcluster, "U16"=w508:u16, "Bytes out"=w509:string)  [unwired: 6 in]
          n163 = Bundle By Name(cluster=w507, "Module Type Code"=w508) -> (w513:T1)
        }
        frame "mod_fpga_ver" {
          n164 = Unbundle By Name(w516) -> ("Module FPGA Version"=w515:u16)
          n165 = call-poly "Becker-Hickl Read Single Data.vi"("Error In"=w520, "Default"=w515, "Bytes in"=w521) -> ("Error Out"=w519:errorcluster, "U16"=w517:u16, "Bytes out"=w518:string)  [unwired: 6 in]
          n166 = Bundle By Name(cluster=w516, "Module FPGA Version"=w517) -> (w522:T1)
        }
        frame "overflow_corr_factor" {
          n167 = Unbundle By Name(w525) -> ("Overflow Corr Factor"=w524:sgl)
          n168 = call-poly "Becker-Hickl Read Single Data.vi"("Error In"=w529, "Default"=w524, "Bytes in"=w530) -> ("Error Out"=w528:errorcluster, "SGL"=w526:sgl, "Bytes out"=w527:string)  [unwired: 6 in]
          n169 = Bundle By Name(cluster=w525, "Overflow Corr Factor"=w526) -> (w531:T1)
        }
        frame "adc_zoom" {
          n170 = Unbundle By Name(w534) -> ("ADC Zoom"=w533:i32)
          n171 = call-poly "Becker-Hickl Read Single Data.vi"("Error In"=w538, "Default"=w533, "Bytes in"=w539) -> ("Error Out"=w537:errorcluster, "I32"=w535:i32, "Bytes out"=w536:string)  [unwired: 6 in]
          n172 = Bundle By Name(cluster=w534, "ADC Zoom"=w535) -> (w540:T1)
        }
        frame "cycles" {
          n173 = Unbundle By Name(w543) -> ("Cycles"=w542:i32)
          n174 = call-poly "Becker-Hickl Read Single Data.vi"("Error In"=w547, "Default"=w542, "Bytes in"=w548) -> ("Error Out"=w546:errorcluster, "I32"=w544:i32, "Bytes out"=w545:string)  [unwired: 6 in]
          n175 = Bundle By Name(cluster=w543, "Cycles"=w544) -> (w549:T1)
        }
        frame "StopInfo" {
          n176 = Unbundle By Name(w557) -> ("Measurement Stop Info"=w552:T2)
          n177 = call "Load Becker-Hickl Measurement Stop Information.vi"("error in (no error)"=w554, "Measurement Stop Info in"=w552, "string in"=w556) -> ("error out"=w553:errorcluster, "Measurement Stop Info out"=w551:T2, "string out"=w555:string)  [unwired: 6 in]
          n178 = Bundle By Name(cluster=w557, "Measurement Stop Info"=w551) -> (w558:T1)
        }
        frame "FCSInfo" {
          n179 = Unbundle By Name(w566) -> ("Measurement FCS Info"=w561:T3)
          n180 = call "Load Becker-Hickl Measurement FCS Information.vi"("error in (no error)"=w563, "Measurement FCS Info in"=w561, "string in"=w565) -> ("error out"=w562:errorcluster, "Measurement FCS Info out"=w560:T3, "string out"=w564:string)  [unwired: 6 in]
          n181 = Bundle By Name(cluster=w566, "Measurement FCS Info"=w560) -> (w567:T1)
        }
        frame "image_x" {
          n182 = Unbundle By Name(w570) -> ("Image X"=w569:i32)
          n183 = call-poly "Becker-Hickl Read Single Data.vi"("Error In"=w574, "Default"=w569, "Bytes in"=w575) -> ("Error Out"=w573:errorcluster, "I32"=w571:i32, "Bytes out"=w572:string)  [unwired: 6 in]
          n184 = Bundle By Name(cluster=w570, "Image X"=w571) -> (w576:T1)
        }
        frame "image_y" {
          n185 = Unbundle By Name(w579) -> ("Image Y"=w578:i32)
          n186 = call-poly "Becker-Hickl Read Single Data.vi"("Error In"=w583, "Default"=w578, "Bytes in"=w584) -> ("Error Out"=w582:errorcluster, "I32"=w580:i32, "Bytes out"=w581:string)  [unwired: 6 in]
          n187 = Bundle By Name(cluster=w579, "Image Y"=w580) -> (w585:T1)
        }
        frame "image_rx" {
          n188 = Unbundle By Name(w588) -> ("Image RX"=w587:i32)
          n189 = call-poly "Becker-Hickl Read Single Data.vi"("Error In"=w592, "Default"=w587, "Bytes in"=w593) -> ("Error Out"=w591:errorcluster, "I32"=w589:i32, "Bytes out"=w590:string)  [unwired: 6 in]
          n190 = Bundle By Name(cluster=w588, "Image RX"=w589) -> (w594:T1)
        }
        frame "image_ry" {
          n191 = Unbundle By Name(w597) -> ("Image RY"=w596:i32)
          n192 = call-poly "Becker-Hickl Read Single Data.vi"("Error In"=w601, "Default"=w596, "Bytes in"=w602) -> ("Error Out"=w600:errorcluster, "I32"=w598:i32, "Bytes out"=w599:string)  [unwired: 6 in]
          n193 = Bundle By Name(cluster=w597, "Image RY"=w598) -> (w603:T1)
        }
        frame "xy_gain" {
          n194 = Unbundle By Name(w606) -> ("XY Gain"=w605:i16)
          n195 = call-poly "Becker-Hickl Read Single Data.vi"("Error In"=w610, "Default"=w605, "Bytes in"=w611) -> ("Error Out"=w609:errorcluster, "I16"=w607:i16, "Bytes out"=w608:string)  [unwired: 6 in]
          n196 = Bundle By Name(cluster=w606, "XY Gain"=w607) -> (w612:T1)
        }
        frame "master_clock" {
          n197 = Unbundle By Name(w615) -> ("Master Clock"=w614:i16)
          n198 = call-poly "Becker-Hickl Read Single Data.vi"("Error In"=w619, "Default"=w614, "Bytes in"=w620) -> ("Error Out"=w618:errorcluster, "I16"=w616:i16, "Bytes out"=w617:string)  [unwired: 6 in]
          n199 = Bundle By Name(cluster=w615, "Master Clock"=w616) -> (w621:T1)
        }
        frame "adc_de" {
          n200 = Unbundle By Name(w624) -> ("ADC Delay"=w623:i16)
          n201 = call-poly "Becker-Hickl Read Single Data.vi"("Error In"=w628, "Default"=w623, "Bytes in"=w629) -> ("Error Out"=w627:errorcluster, "I16"=w625:i16, "Bytes out"=w626:string)  [unwired: 6 in]
          n202 = Bundle By Name(cluster=w624, "ADC Delay"=w625) -> (w630:T1)
        }
        frame "det_type" {
          n203 = Unbundle By Name(w633) -> ("Detector Type"=w632:i16)
          n204 = call-poly "Becker-Hickl Read Single Data.vi"("Error In"=w637, "Default"=w632, "Bytes in"=w638) -> ("Error Out"=w636:errorcluster, "I16"=w634:i16, "Bytes out"=w635:string)  [unwired: 6 in]
          n205 = Bundle By Name(cluster=w633, "Detector Type"=w634) -> (w639:T1)
        }
        frame "x_axis" {
          n206 = Unbundle By Name(w642) -> ("X Axis"=w641:i16)
          n207 = call-poly "Becker-Hickl Read Single Data.vi"("Error In"=w646, "Default"=w641, "Bytes in"=w647) -> ("Error Out"=w645:errorcluster, "I16"=w643:i16, "Bytes out"=w644:string)  [unwired: 6 in]
          n208 = Bundle By Name(cluster=w642, "X Axis"=w643) -> (w648:T1)
        }
        frame "HISTInfo" {
          n209 = Unbundle By Name(w657) -> ("Addl Histogram Measurement Info"=w651:T4)
          n210 = call "Load Becker-Hickl Measurement Histo Information.vi"("error in (no error)"=w654, "Measurement FCS Info in"=w651, "string in"=w655) -> ("error out"=w652:errorcluster, "Measurement FCS Info out"=w650:T4, "string out"=w653:string)  [unwired: 6 in]
          n211 = Bundle By Name(cluster=w657, "Addl Histogram Measurement Info"=w650) -> (w658:T1)
        }
      }
    }
  }
  "Measurement Information" <- w1
  n212 = Close File(refnum=w8, error in=w7) -> (path=→"File Path":path, error out=→"Error Out":errorcluster)
